vi "OAT Easy Resample Spectral Map.vi"   [LabVIEW 2017]
doc: "Computes the spectral map of <B>scaled signal [EU]</B> based on the resampling method. You can use this polymorphic VI to obtain a spectral map for an analog tachometer signal or a digital tachometer signal. The data type you wire to the <B>analog tach signal</B> input determines the polymorphic instance to use."
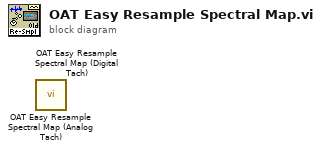
[diagram p0: block diagram]
diagram:
  n1 = call <vilib>:"OAT Easy Resample Spectral Map (Analog Tach).vi"() -> ()  [unwired: 11 in, 5 out]
  n2 = call <vilib>:"OAT Easy Resample Spectral Map (Digital Tach).vi"() -> ()  [unwired: 11 in, 5 out]
